vi "Initialize.vi"(0 "VISA resource name":refnum<visa-resource-name>, 7 "ID Query (T: Check)":bool=TRUE, 9 "Reset (T: Reset)":bool=TRUE, 11 "error in (no error)":errorcluster) -> (4 "VISA resource name out":refnum<visa-resource-name>, 6 "Instrument ID":string, 15 "error out":errorcluster)   [LabVIEW 2019, in "Yokogawa WT200 Series.lvlib"]
doc: "This VI passes the addressing information in the instrument descriptor to the Instr Open VI and returns the instrument ID. You can optionally reset the instrument by setting the front panel reset control. You must run this VI before using any of the instrument driver VIs for this instrument.\n\nNote : All parameters of ASRLx interface are stored to the \"visaconf.ini\" file. To configure serial interface use please T&M Explorer or Measurement & Automation Explorer. And the terminator is set to \"LF\".\n This insturument driver use the communication commands conforming to the IEEE 488.2 Standard."
uses:
  Yokogawa WT200 Series.lvlib
panel:
  # "© 2005 National Instruments.  ALL RIGHTS RESERVED."
  # "Check\nDon't Check"
  # "Reset\nDon't Reset"
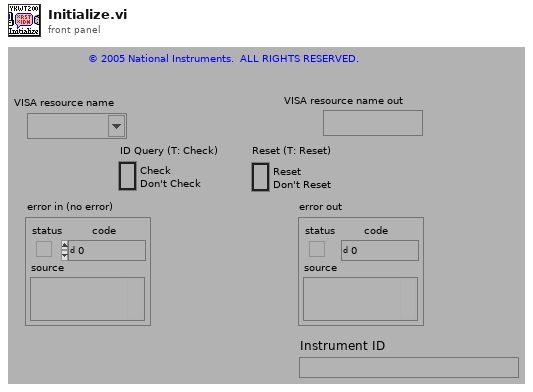
[diagram p1: front panel]
types:
  T1 = cluster{"status":bool, "code":i32, "VI name":string}
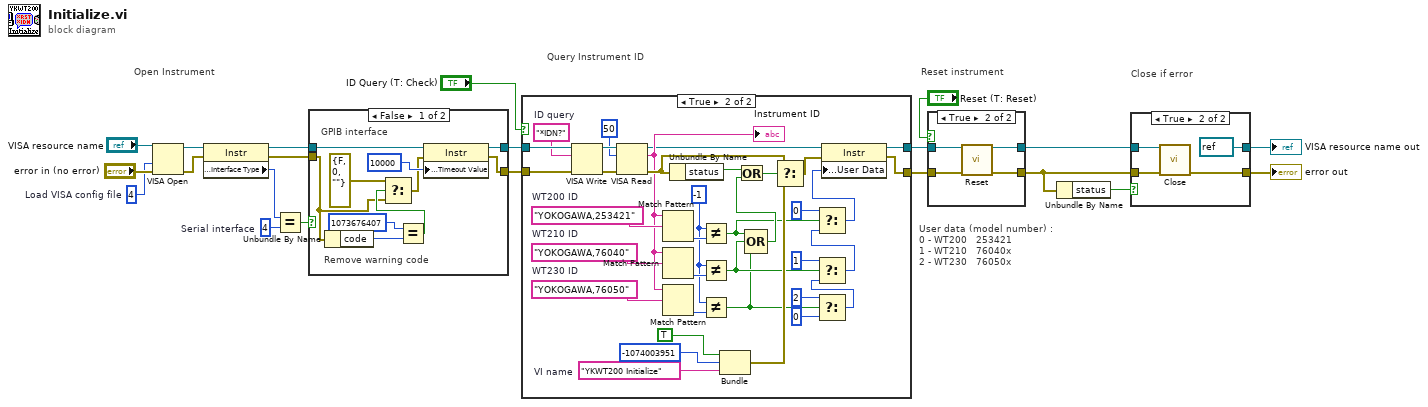
[diagram p0: block diagram]
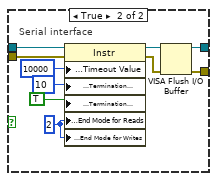
[diagram p2: hidden frame]
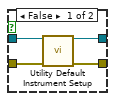
[diagram p4: hidden frame]
diagram:
  w2 = u16 4  # Serial interface
  w9 = u32 4  # Load VISA config file
  # "User data (model number) : \n0 - WT200   253421\n1 - WT210   76040x\n2 - WT230   76050x"
  # "Close if error"
  # "Query Instrument ID"
  # "Reset instrument"
  # "Open Instrument"
  n1 = VISA Open(access mode=w9, error in (no error)="error in (no error)", VISA resource name="VISA resource name") -> (VISA resource name=w8:refnum<visa-resource-name>, error out=w7:errorcluster)  [unwired: 2 in]
  n2 = property class="Instr"(reference=w8, error in=w7) -> (reference out=w6:refnum<visa-resource-name>, error out=w5:errorcluster, "Interface Information:Interface Type"=w3:u16)
  n3 = Equal?(x=w3, y=w2) -> (x = y?=w4:bool)
  n4 = case shown="False" w4 {
    tunnel: [w31 w33] -> w11
    tunnel: [w30 w32] -> w10
    tunnel: w6 -> [w29 w37]
    tunnel: w5 -> [w24 w36]
    frame False {
      # "GPIB interface"
      # "Remove warning code"
      n5 = Unbundle By Name(w24) -> ("code"=w27:i32)
      n6 = Equal?(x=1073676407, y=w27) -> (x = y?=w25:bool)
      n7 = Select(t=errorcluster {"status"=FALSE, "code"=0, "source"=""}, s=w25, f=w24) -> (s? t:f=w22:errorcluster)
      n8 = property class="Instr"(reference=w29, error in=w22, "General Settings:Timeout Value"=u32 10000 ("Tmo Value")) -> (reference out=w31:refnum<visa-resource-name>, error out=w30:errorcluster)
    }
    frame True {
      w38 = u16 2
      # "Serial interface"
      n9 = property class="Instr"(reference=w37, error in=w36, "General Settings:Timeout Value"=u32 10000 ("Tmo Value"), "Message Based Settings:Termination Character"=u8 10, "Message Based Settings:Termination Character Enable"=TRUE, "Serial Settings:End Mode for Reads"=w38, "Serial Settings:End Mode for Writes"=w38) -> (reference out=w35:refnum<visa-resource-name>, error out=w34:errorcluster)
      n10 = VISA Flush I/O Buffer(VISA resource name=w35, error in (no error)=w34) -> (VISA resource name out=w33:refnum<visa-resource-name>, error out=w32:errorcluster)  [unwired: 1 in]
    }
  }
  n11 = case shown="True" "ID Query (T: Check)" {
    tunnel: [w42 w54] -> w20
    tunnel: [w43 w55] -> w21
    tunnel: w11 -> [w43 w75]
    tunnel: w10 -> [w42 w74]
    frame False {
    }
    frame True {
      w62 = "YOKOGAWA,76050"  # WT230 ID
      w64 = "YOKOGAWA,76040"  # WT210 ID
      w65 = "YOKOGAWA,253421"  # WT200 ID
      w70 = "YKWT200 Initialize"  # VI name
      w59 = -1
      w73 = "*IDN?"  # ID query
      n12 = VISA Write(VISA resource name=w75, write buffer=w73, error in (no error)=w74) -> (VISA resource name out=w76:refnum<visa-resource-name>, error out=w79:errorcluster)  [unwired: 1 out]
      n13 = VISA Read(VISA resource name=w76, byte count=u32 50, error in (no error)=w79) -> (VISA resource name out=w57:refnum<visa-resource-name>, read buffer=w60:string, error out=w67:errorcluster)  [unwired: 1 out]
      "Instrument ID" <- w60
      n14 = Match Pattern(string=w60, regular expression=w65) -> (offset past match=w71:i32)  [unwired: 1 in, 3 out]
      n15 = Match Pattern(string=w60, regular expression=w64) -> (offset past match=w63:i32)  [unwired: 1 in, 3 out]
      n16 = Match Pattern(string=w60, regular expression=w62) -> (offset past match=w61:i32)  [unwired: 1 in, 3 out]
      n17 = Unbundle By Name(w67) -> ("status"=w66:bool)
      n18 = Not Equal?(x=w59, y=w71) -> (x != y?=w47:bool)
      n19 = Not Equal?(x=w59, y=w63) -> (x != y?=w53:bool)
      n20 = Not Equal?(x=w59, y=w61) -> (x != y?=w52:bool)
      n21 = Bundle(TRUE, -1074003951, "VI name"=w70) -> (w77:cluster{bool, i32, "VI name":string})  [unwired: 1 in]
      n22 = Compound Arithmetic op=OR(w47, w53, w52) -> (w58:bool)
      n23 = Or(x=w66, y=w58) -> (x .or. y?=w68:bool)
      n24 = Select(t=w67, s=w68, f=w77) -> (s? t:f=w56:T1)
      n25 = Select(t=u32 2, s=w52, f=u32 0) -> (s? t:f=w49:u32)
      n26 = Select(t=u32 1, s=w53, f=w49) -> (s? t:f=w46:u32)
      n27 = Select(t=u32 0, s=w47, f=w46) -> (s? t:f=w44:u32)
      n28 = property class="Instr"(reference=w57, error in=w56, "General Settings:User Data"=w44) -> (reference out=w55:refnum<visa-resource-name>, error out=w54:errorcluster)
    }
  }
  n29 = case shown="True" "Reset (T: Reset)" {
    tunnel: w20 -> [w82 w87]
    tunnel: [w83 w86] -> w13
    tunnel: w21 -> [w81 w84]
    tunnel: [w80 w85] -> w16
    frame False {
      n30 = call "Utility Default Instrument Setup.vi"("VISA resource name"=w81, "error in (no error)"=w82) -> ("VISA resource name out"=w80:refnum<visa-resource-name>, "error out"=w83:errorcluster)  [unwired: 12 in]
    }
    frame True {
      n31 = call "Reset.vi"("VISA resource name"=w84, "error in (no error)"=w87) -> ("VISA resource name out"=w85:refnum<visa-resource-name>, "error out"=w86:errorcluster)  [unwired: 12 in]
    }
  }
  n32 = Unbundle By Name(w13) -> ("status"=w12:bool)
  n33 = case shown="True" w12 {
    tunnel: w13 -> [w88 w93]
    tunnel: w16 -> [w89 w92]
    tunnel: [w89 refnum<visa-resource-name> refnum ("VISA resource name out")] -> w15
    tunnel: [w88 w91] -> w14
    frame False {
    }
    frame True {
      n34 = call "Close.vi"("VISA resource name"=w92, "error in (no error)"=w93) -> ("error out"=w91:errorcluster)  [unwired: 13 in]
    }
  }
  "VISA resource name out" <- w15
  "error out" <- w14
